vi "Post-Process.vi"(11 "Zap Sat in":refnum<class "Zap Sat.lvclass">) -> (2 "New Elements":refnum<class "Element.lvclass">[](array[class]), 3 "Zap Sat out":refnum<class "Zap Sat.lvclass">)   [LabVIEW 2021, in "Zap Sat.lvclass"]
uses:
  Zap Sat.lvclass
  Element/Element.lvclass
  Weapons/Laser/Laser.lvclass
  C:/dev/LabVIEW/LabMelee/Source/Application Specific/Element/Element.lvclass
  Deployable/Deployable.lvclass
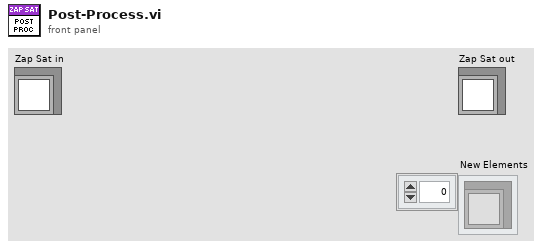
[diagram p1: front panel]
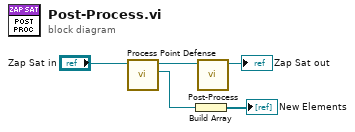
[diagram p0: block diagram]
diagram:
  n1 = call "Process Point Defense.vi"("Deployable in"="Zap Sat in") -> ("Laser out"=w2:refnum<class "Laser.lvclass">, "Deployable out"=w3:refnum<class "Zap Sat.lvclass">)  [unwired: 9 in]
  n2 = Build Array(w2) -> (→"New Elements":refnum<class "Laser.lvclass">[])
  n3 = call-parent "Post-Process.vi"("Element in"=w3) -> ("Element out"=→"Zap Sat out":refnum<class "Zap Sat.lvclass">)  [unwired: 9 in, 1 out]
